vi "Utility Voltage Setting Mode.vi"(0 "VISA resource name":refnum<visa-resource-name>, 11 "error in (no error)":errorcluster) -> (4 "VISA resource name out":refnum<visa-resource-name>, 8 "Query Response":string, 15 "error out":errorcluster {"code" format="%.0x"})   [LabVIEW 2010, in "Stanford Research PS300 Series.lvlib"]
doc: "This VI queries for the voltage setting mode. The setting mode can be controlled either by the front panel or the rear panel\n\nNotes*: The rear setting mode can be changed only when the rear panel VOLTAGE switch is on SET mode."
uses:
  <instrlib>/Stanford Research PS300 Series/Stanford Research PS300 Series.lvlib
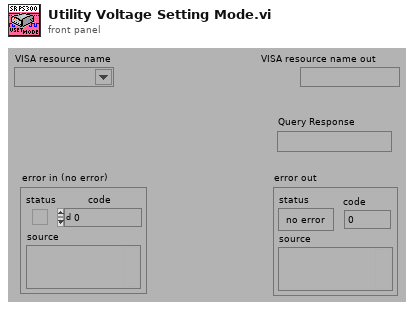
[diagram p1: front panel]
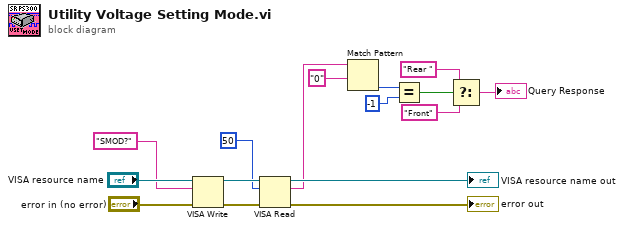
[diagram p0: block diagram]
diagram:
  n1 = VISA Write(VISA resource name="VISA resource name", write buffer="SMOD?", error in (no error)="error in (no error)") -> (VISA resource name out=w13:refnum<visa-resource-name>, error out=w12:errorcluster)  [unwired: 1 out]
  n2 = VISA Read(VISA resource name=w13, byte count=u32 50 ("byte count (0)"), error in (no error)=w12) -> (VISA resource name out=→"VISA resource name out":refnum<visa-resource-name>, read buffer=w9:string, error out=→"error out":errorcluster)  [unwired: 1 out]
  n3 = Match Pattern(string=w9, regular expression="0") -> (offset past match=w7:i32)  [unwired: 1 in, 3 out]
  n4 = Equal?(x=w7, y=-1) -> (x = y?=w5:bool)
  n5 = Select(t="Rear ", s=w5, f="Front") -> (s? t:f=→"Query Response":string)
